vi "Prepare Command.vi"(8 "error in":errorcluster, 11 "CIFCorePlugin in":refnum<class "CIFCorePlugin.lvclass">) -> (0 "error out":errorcluster, 3 "CIFCorePlugin out":refnum<class "CIFCorePlugin.lvclass">)   [LabVIEW 2021, in "CIFCorePlugin.lvclass"]
uses:
  CIFCorePlugin.lvclass
  CIFCorePlugin.lvclass/CIFCorePlugin.ctl
  Typedef/gRPC to Main Command Payload.ctl
  Typedef/gRPC to Main Commands.ctl
  0124de93-67bc-4437-967e-5a501b30d5f0.vi
  <vilib>/CIF Foundation/CIF CIPC/SubVIs/Check Error.vi
  <vilib>/CIF Foundation/CIF CIPC/SubVIs/Notify Of New Write.vi
  <vilib>/CIF Foundation/CIF CIPC/SubVIs/Get dll Path.vi
  <vilib>/CIF Foundation/CIF CIPC/SubVIs/Get Element Write Position.vi
  <vilib>/CIF Foundation/CIF CIPC/SubVIs/Get Element Info Variant.vi
  <vilib>/Utility/error.llb/Trim Whitespace.vi
  <vilib>/Utility/error.llb/Error Cluster From Error Code.vi
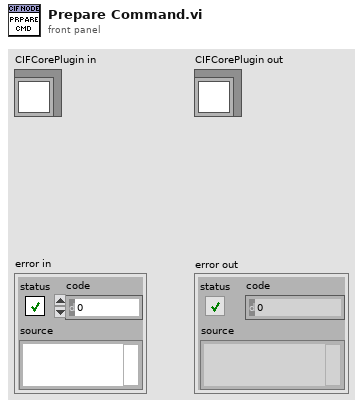
[diagram p1: front panel]
types:
  T1 = typedef "CIFCorePlugin.lvclass/gRPC to Main Command Payload.ctl" = cluster{"OOB_Rx Command":T2, "Array Index":i32}
  T2 = typedef "CIFCorePlugin.lvclass/gRPC to Main Commands.ctl" = enum8{"Start", "Pause", "Stop", "RefreshStats", "UpdateConfig", "Update Clock Map", "Connect Channel", "Force Channel", "Add Publisher Instance", "Remove Publisher Instance", "Prepare"}
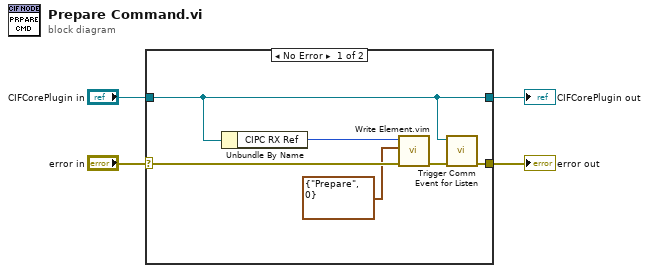
[diagram p0: block diagram]
diagram:
  n1 = case shown="No Error" "error in" {
    selector: "error in" -> [w10 w12]
    tunnel: [w6 w12] -> w3
    tunnel: "CIFCorePlugin in" -> [w5 w11]
    tunnel: [w5 w11] -> w1
    frame No Error {
      n2 = Unbundle By Name(w5) -> ("CIPC RX Ref"=w9:u64)
      n3 = call "Write Element.vim"("error in (no error)"=w10, "Data in"=T1 {"OOB_Rx Command"=enum."Prepare", "Array Index"=0} ("gRCP to Main Command Payload"), "CIPC Reference in"=w9) -> ("error out"=w7:errorcluster)  [unwired: 5 in, 3 out]
      n4 = call "Trigger Comm Event for Listen.vi"("error in (no error)"=w7, "CIFCorePlugin in"=w5) -> ("error out"=w6:errorcluster)  [unwired: 9 in]
    }
    frame Error {
    }
  }
  "error out" <- w3
  "CIFCorePlugin out" <- w1
